vi "HandleFlushAck.vi"(8 "error in (no error)":errorcluster, 11 "LogManager in":refnum<class "LogManager.lvclass">) -> (0 "error out":errorcluster, 3 "LogManager out":refnum<class "LogManager.lvclass">)   [LabVIEW 2026, in "Lumberjack.lvlib" / "LogManager.lvclass"]
doc: "Handle one appender's flush ack during shutdown drain: decrement pendingFlushCount; when it hits 0 while draining, send the manager its own Normal Stop (selfEnqueuer) so the tree stops only after every appender has flushed. No-op when not draining. Community (called by FlushAckMsg)."
uses:
  LogManager.lvclass
  LogManager.lvclass/LogManager.ctl
  <vilib>/ActorFramework/Message Enqueuer/Message Enqueuer.lvclass/Message Enqueuer.ctl
  <vilib>/ActorFramework/Message Enqueuer/Enqueue.vi
  <vilib>/ActorFramework/Stop Msg/Stop Msg.lvclass
  <vilib>/ActorFramework/Message Priority Queue/Priority Enqueue.vi
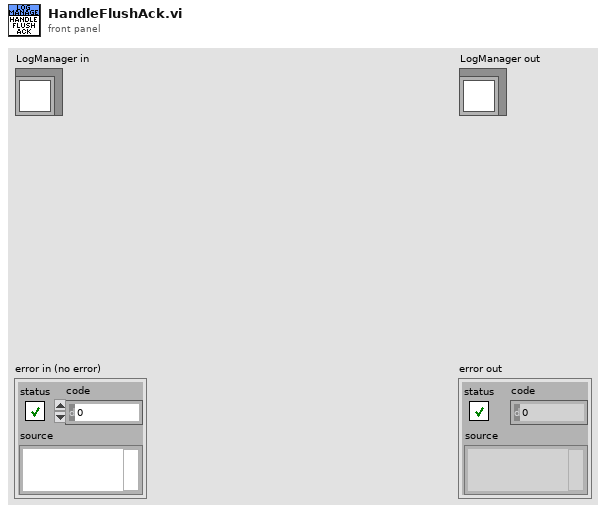
[diagram p1: front panel]
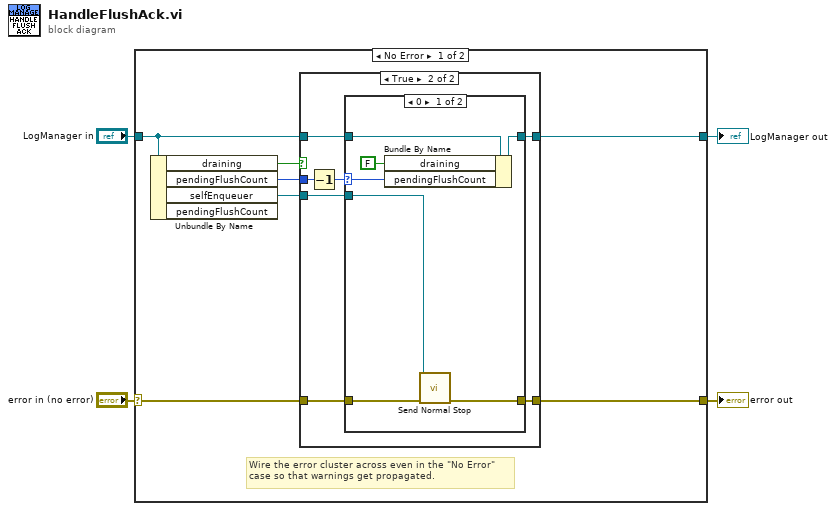
[diagram p0: block diagram]
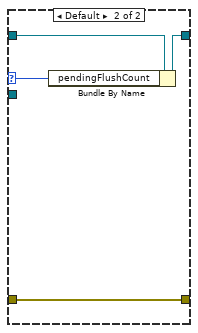
[diagram p3: hidden frame]
diagram:
  n1 = case shown="No Error" "error in (no error)" {
    selector: "error in (no error)" -> [w6 w33]
    tunnel: [w5 w33] -> w3
    tunnel: [w9 w32] -> w1
    tunnel: "LogManager in" -> [w10 w32]
    frame No Error {
      # "Wire the error cluster across even in the \"No Error\"\ncase so that warnings get propagated."
      n2 = Unbundle By Name(w10) -> ("draining"=w11:bool, "pendingFlushCount"=w7:i32, "selfEnqueuer"=w8:refnum<class "Message Enqueuer.lvclass">)  [unwired: 1 out]
      n3 = case shown="True" w11 {
        tunnel: w10 -> [w13 w18]
        tunnel: w6 -> [w12 w16]
        tunnel: [w13 w17] -> w9
        tunnel: [w12 w15] -> w5
        tunnel: w7 -> [_ w20]
        tunnel: w8 -> [_ w14]
        frame False {
        }
        frame True {
          n4 = Decrement(x=w20) -> (x-1=w19:i32)
          n5 = case shown="0" w19 {
            selector: w19 -> [w22 w28]
            tunnel: w18 -> [w27 w31]
            tunnel: [w26 w30] -> w17
            tunnel: w16 -> [w25 w29]
            tunnel: [w21 w29] -> w15
            tunnel: w14 -> [w24 _]
            frame 0 {
              n6 = Bundle By Name(cluster=w27, "draining"=FALSE, "pendingFlushCount"=w22) -> (w26:refnum<class "LogManager.lvclass">)
              n7 = call <vilib>:"Send Normal Stop.vi"("error in (no error)"=w25, "Message Enqueuer"=w24) -> ("error out"=w21:errorcluster)  [unwired: 9 in]
            }
            frame Default {
              n8 = Bundle By Name(cluster=w31, "pendingFlushCount"=w28) -> (w30:refnum<class "LogManager.lvclass">)
            }
          }
        }
      }
    }
    frame Error {
    }
  }
  "error out" <- w3
  "LogManager out" <- w1
